vi "Save VI Hierarchy.vi"(8 "error in (no error)":errorcluster, 10 "Current VI's Path":path, 11 "Path to the Top Level VI Causing the Issue":path) -> (0 "error out":errorcluster, 1 "Top Level Path":path, 2 "Destination Directory":path, 4 "Zip File Name":string)   [LabVIEW 2014, in "Raspberry Pi Compatible Compiler for LabVIEW.lvlib"]
uses:
  Raspberry Pi Compatible Compiler for LabVIEW.lvlib
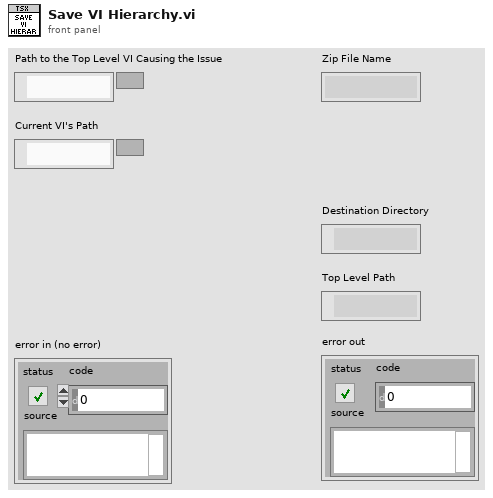
[diagram p1: front panel]
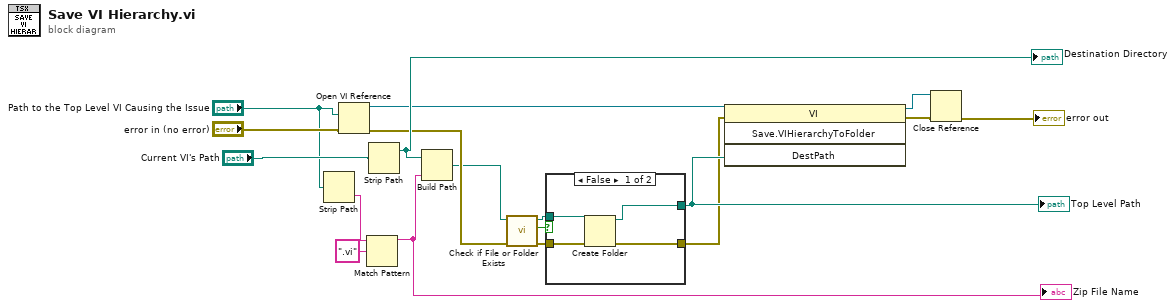
[diagram p0: block diagram]
diagram:
  n1 = Strip Path(path="Path to the Top Level VI Causing the Issue") -> (name=w7:string)  [unwired: 1 out]
  n2 = Open VI Reference(vi path="Path to the Top Level VI Causing the Issue", error in (no error)="error in (no error)") -> (vi reference=w6:refnum<vi>, error out=w11:errorcluster)  [unwired: 4 in]
  n3 = Match Pattern(string=w7, regular expression=".vi") -> (before substring=w15:string)  [unwired: 1 in, 3 out]
  "Zip File Name" <- w15
  n4 = Strip Path(path="Current VI's Path") -> (stripped path=w16:path)  [unwired: 1 out]
  "Destination Directory" <- w16
  n5 = Build Path(base path=w16, name or relative path=w15) -> (appended path=w9:path)
  n6 = call <vilib>:"Check if File or Folder Exists.vi"("error in (no error)"=w11, "path"=w9) -> ("error out"=w13:errorcluster, "file or folder exists?"=w10:bool, "dup path"=w12:path)  [unwired: 7 in]
  n7 = case shown="False" w10 {
    tunnel: w12 -> [w22 w24]
    tunnel: w13 -> [w21 w23]
    tunnel: [w20 w24] -> w17
    tunnel: [w19 w23] -> w14
    frame False {
      n8 = Create Folder(path (use dialog)=w22, error in=w21) -> (created path=w20:path, error out=w19:errorcluster)  [unwired: 1 in, 1 out]
    }
    frame True {
    }
  }
  "Top Level Path" <- w17
  n9 = invoke class="VI" method="Save.VIHierarchyToFolder"(reference=w6, error in=w14, "DestPath"=w17) -> (reference out=w1:refnum<vi>, error out=w3:errorcluster)  [unwired: 1 in, 2 out]
  n10 = Close Reference(reference=w1, error in (no error)=w3) -> (error out=→"error out":errorcluster)
